vi "Write Log File Header.vi"(8 "error in (no error)":errorcluster, 10 "Header Text":string, 11 "Text Log File in":refnum<class "Text Log File.lvclass">) -> (0 "error out":errorcluster, 3 "Text Log File out":refnum<class "Text Log File.lvclass">)   [LabVIEW 2015, in "Text Log File.lvclass"]
doc: "Write the text file header information, including custom header text."
uses:
  Text Log File.lvclass
  Text Log File.lvclass/Text Log File.ctl
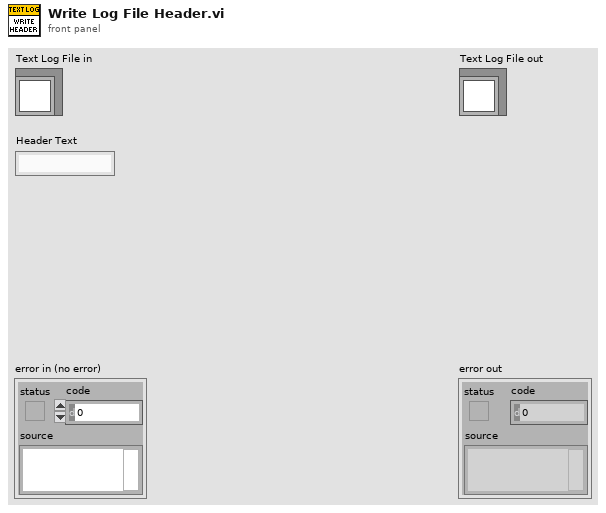
[diagram p1: front panel]
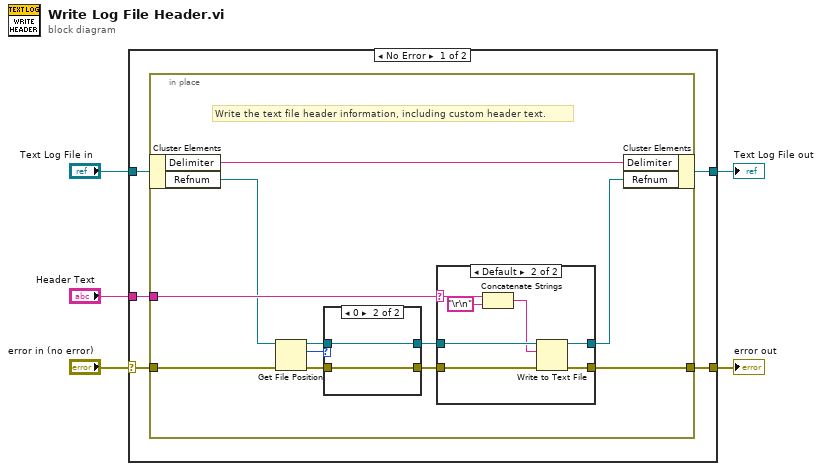
[diagram p0: block diagram]
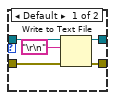
[diagram p2: hidden frame]
diagram:
  n1 = case shown="No Error" "error in (no error)" {
    selector: "error in (no error)" -> [w6 w38]
    tunnel: "Text Log File in" -> [w10 w39]
    tunnel: [w9 w39] -> w4
    tunnel: [w8 w38] -> w3
    tunnel: "Header Text" -> [w7 _]
    frame No Error {
      n2 = in-place {
        in-place-border: w6 -> [w20]
        in-place-border: [w11] -> w8
        in-place-border: w7 -> [w21]
        # "Write the text file header information, including custom header text."
        n3 = in-place-cluster #1(w10) -> ("Delimiter"=w19:string, "Refnum"=w18:refnum<file>)
        n4 = Get File Position(4:w20, 7:w18) -> (0:w13:errorcluster, 2:w17:i64, 3:w15:refnum<file>)
        n5 = case shown="0" w17 {
          tunnel: [w24 w28] -> w16
          tunnel: w15 -> [w26 w28]
          tunnel: [w23 w27] -> w14
          tunnel: w13 -> [w25 w27]
          frame Default {
            n6 = Write to Text File(file (use dialog)=w26, text="\r\n", error in=w25) -> (refnum out=w24:refnum<file>, error out=w23:errorcluster)  [unwired: 1 in, 1 out]
          }
          frame 0 {
          }
        }
        n7 = case shown="Default" w21 {
          selector: w21 -> [_ w35]
          tunnel: w14 -> [w30 w34]
          tunnel: [w30 w33] -> w11
          tunnel: w16 -> [w29 w37]
          tunnel: [w29 w36] -> w12
          frame "" {
            # "No header text specified."
          }
          frame Default {
            n8 = Concatenate Strings(w35, "\r\n") -> (w32:string)
            n9 = Write to Text File(file (use dialog)=w37, text=w32, error in=w34) -> (refnum out=w36:refnum<file>, error out=w33:errorcluster)  [unwired: 1 in, 1 out]
          }
        }
        n10 = in-place-cluster #1("Delimiter"=w19, "Refnum"=w12) -> (w9:refnum<class "Text Log File.lvclass">)
      }
    }
    frame Error {
    }
  }
  "error out" <- w3
  "Text Log File out" <- w4
